vi "GetSpect.vi"(3 "error in (no error)":errorcluster, 5 "SpectRef In":T1) -> (0 "error out":errorcluster, 1 "Spectrum Values":dbl[](array[numeric]), 2 "SpectRef Out":T1)   [LabVIEW 2012]
uses:
  Controls/USB4000_Data.ctl
panel:
  out "appended path 2":path
  out "appended path":path
  out "Length":i32
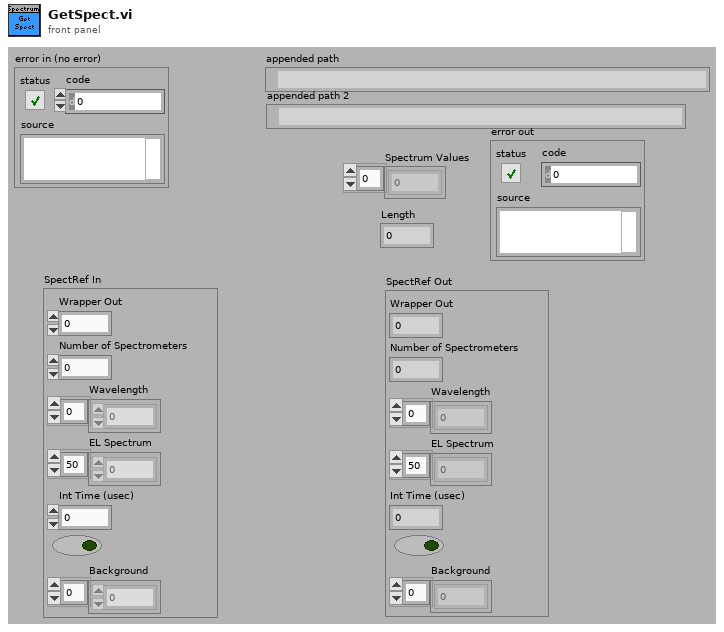
[diagram p1: front panel]
types:
  T1 = typedef "USB4000_Data.ctl" = cluster{"Wrapper Out":u32, "Number of Spectrometers":i32, "Wavelength":dbl[], "EL Spectrum":dbl[], "Int Time (usec)":i32, bool, "Background":dbl[]}
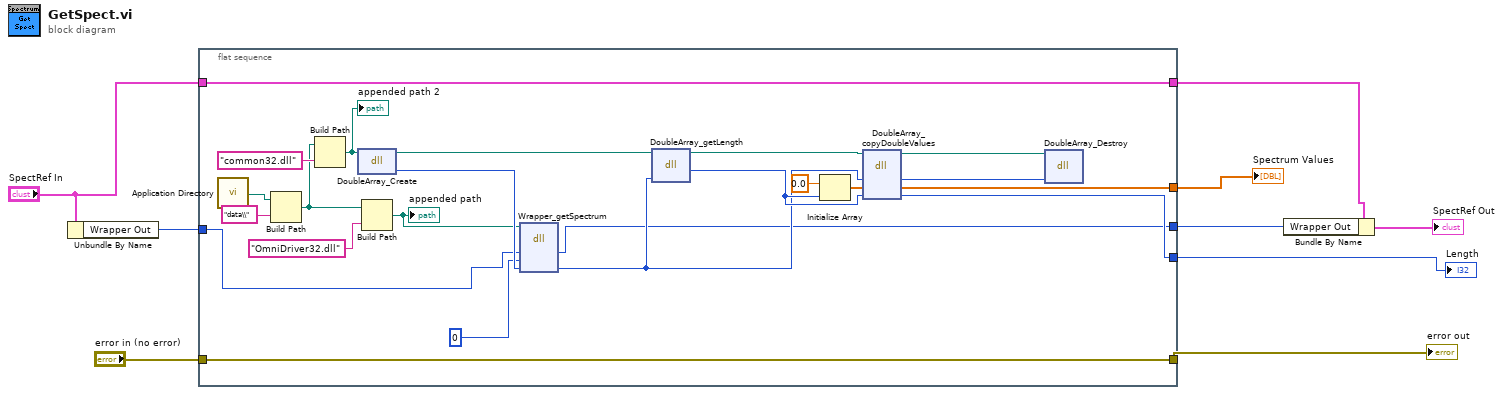
[diagram p0: block diagram]
diagram:
  n1 = Unbundle By Name("SpectRef In") -> ("Wrapper Out"=w5:u32)
  n2 = flat-sequence {
    tunnel: [w16] -> w9
    tunnel: [w15] -> w8
    tunnel: [w14] -> w7
    tunnel: "error in (no error)" -> [w14]
    tunnel: w5 -> [w13]
    tunnel: [w11] -> w2
    tunnel: "SpectRef In" -> [w11]
    tunnel: [w10] -> w1
    frame #0 {
      n3 = call <vilib>:"Application Directory.vi"() -> ("Application Directory"=w23:path)
      n4 = Build Path(base path=w23, name or relative path="data\\") -> (appended path=w19:path)
      n5 = Build Path(base path=w19, name or relative path="common32.dll") -> (appended path=w18:path)
      "appended path 2" <- w18
      n6 = dll-call lib="common32.dll" fn="DoubleArray_Create" label="DoubleArray.Create"(path in=w18) -> (path out=w24:path, "return type"=w32:u32)  [unwired: 2 in, 1 out]
      n7 = Build Path(base path=w19, name or relative path="OmniDriver32.dll") -> (appended path=w17:path)
      "appended path" <- w17
      n8 = dll-call lib="D:/Software Development/EPI Development/BurnIn Testing/Instruments/Drivers/Ocean Optics/OOI_HOME/OmniDriver32.dll" fn="Wrapper_getSpectrum" label="Wrapper.getSpectrum"(path in=w17, "Wrapper"=w13, "Index"=0, "DoubbleArray"=w32) -> ("Wrapper"=w10:u32, "DoubbleArray"=w28:u32)  [unwired: 3 in, 3 out]
      n9 = dll-call lib="common32.dll" fn="DoubleArray_getLength" label="DoubleArray.getLength"(path in=w24, "DoubbleArray"=w28) -> (path out=w25:path, "return type"=w29:i32)  [unwired: 3 in, 1 out]
      n10 = Initialize Array(0.0 ("element"), w29) -> (w30:dbl[])
      n11 = dll-call lib="common32.dll" fn="DoubleArray_copyDoubleValues" label="DoubleArray.copyDoubleValues"(path in=w25, "DoubbleArray"=w28, "Values"=w30, "Length"=w29) -> (path out=w26:path, "DoubbleArray"=w27:u32, "Values"=w16:dbl[], "Length"=w15:i32)  [unwired: 2 in, 2 out]
      n12 = dll-call lib="common32.dll" fn="DoubleArray_Destroy" label="DoubleArray.Destroy"(path in=w26, "DoubleArray"=w27) -> ()  [unwired: 3 in, 3 out]
    }
  }
  n13 = Bundle By Name(cluster=w2, "Wrapper Out"=w1) -> (→"SpectRef Out":T1)
  "Spectrum Values" <- w9
  "Length" <- w8
  "error out" <- w7
